vi "Execute.vi"(8 "error in (no error)":errorcluster, 11 "System in":refnum<class "System.lvclass">) -> (0 "error out":errorcluster, 3 "System out":refnum<class "System.lvclass">)   [LabVIEW 2013, in "System.lvclass"]
uses:
  System.lvclass
  System.lvclass/System.ctl
  Commands/Command/Command.lvclass
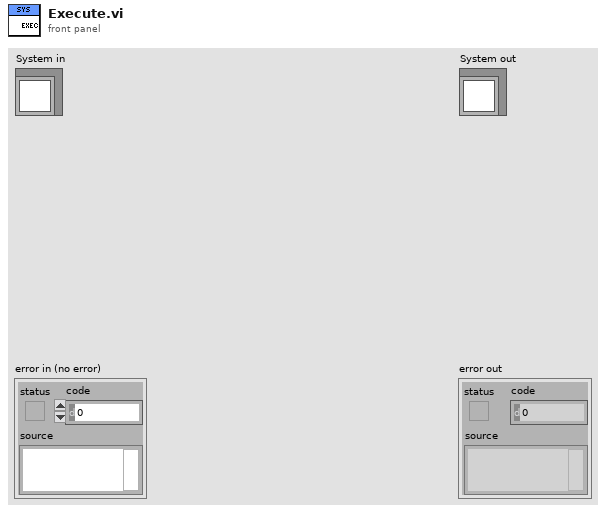
[diagram p1: front panel]
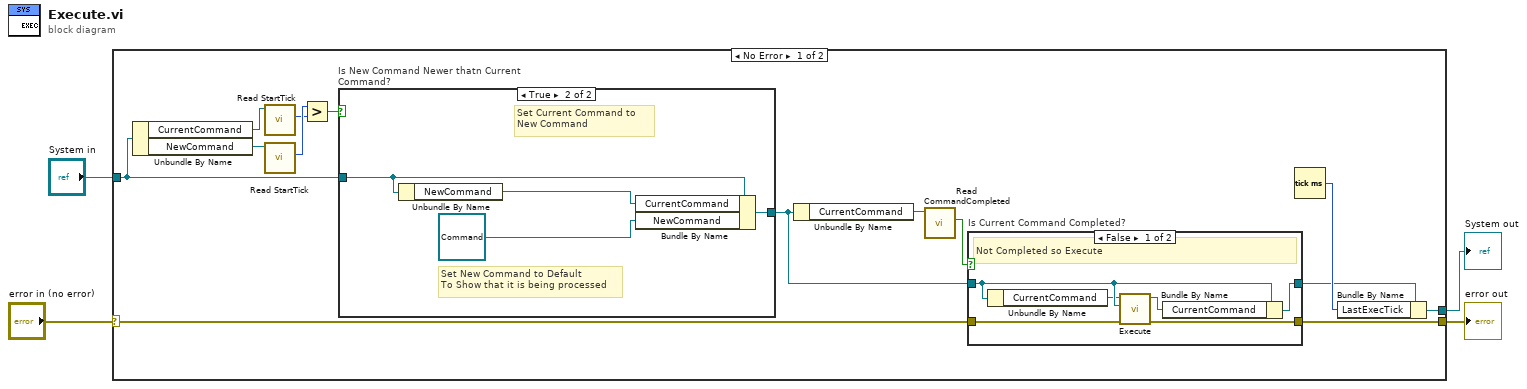
[diagram p0: block diagram]
diagram:
  n1 = case shown="No Error" "error in (no error)" {
    selector: "error in (no error)" -> [w16 w33]
    tunnel: [w17 w33] -> w3
    tunnel: "System in" -> [w6 w32]
    tunnel: [w12 w32] -> w1
    frame No Error {
      n2 = Unbundle By Name(w6) -> ("CurrentCommand"=w11:refnum<class "Command.lvclass">, "NewCommand"=w10:refnum<class "Command.lvclass">)
      n3 = call-dynamic "Read StartTick.vi"("Command in"=w11) -> ("StartTick"=w8:u32)  [unwired: 8 in, 2 out]
      n4 = call-dynamic "Read StartTick.vi"("Command in"=w10) -> ("StartTick"=w9:u32)  [unwired: 8 in, 2 out]
      n5 = Greater?(x=w9, y=w8) -> (0:w7:bool)
      n6 = case "Is New Command Newer thatn Current Command?" shown="True" w7 {
        tunnel: w6 -> [w19 w21]
        tunnel: [w19 w23] -> w5
        frame False {
          # "Don't worry about New Command\nKeep Processing Current Command"
        }
        frame True {
          # "Set New Command to Default\nTo Show that it is being processed"
          # "Set Current Command to \nNew Command"
          n7 = Unbundle By Name(w21) -> ("NewCommand"=w20:refnum<class "Command.lvclass">)
          n8 = Bundle By Name(cluster=w21, "CurrentCommand"=w20, "NewCommand"=refnum<class "Command.lvclass"> refnum ("Command.lvclass")) -> (w23:refnum<class "System.lvclass">)
        }
      }
      n9 = Unbundle By Name(w5) -> ("CurrentCommand"=w15:refnum<class "Command.lvclass">)
      n10 = call-dynamic "Read CommandCompleted.vi"("Command in"=w15) -> ("CommandCompleted"=w14:bool)  [unwired: 8 in, 2 out]
      n11 = case "Is Current Command Completed?" shown="False" w14 {
        tunnel: [w29 w30] -> w17
        tunnel: w16 -> [w28 w30]
        tunnel: w5 -> [w26 w31]
        tunnel: [w27 w31] -> w13
        frame False {
          # "Not Completed so Execute"
          n12 = Unbundle By Name(w26) -> ("CurrentCommand"=w25:refnum<class "Command.lvclass">)
          n13 = call-dynamic "Execute.vi"("error in (no error)"=w28, "System in"=w26, "Command in"=w25) -> ("error out"=w29:errorcluster, "Command out"=w24:refnum<class "Command.lvclass">)  [unwired: 7 in]
          n14 = Bundle By Name(cluster=w26, "CurrentCommand"=w24) -> (w27:refnum<class "System.lvclass">)
        }
        frame True {
          # "Command Completed, Don't Execute"
        }
      }
      n15 = Tick Count (ms)() -> (millisecond timer value=w18:u32)
      n16 = Bundle By Name(cluster=w13, "LastExecTick"=w18) -> (w12:refnum<class "System.lvclass">)
    }
    frame Error {
    }
  }
  "error out" <- w3
  "System out" <- w1
